vi "Orleen.vi"() -> ()   [LabVIEW 2016]
panel:
  out "String 2":string
  out "Numeric":dbl
  in  "String":string
  in  "?":dbl
  in  "?":dbl
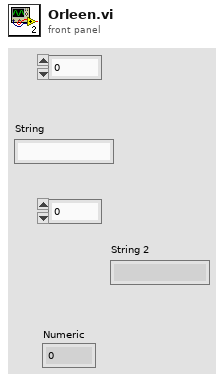
[diagram p1: front panel]
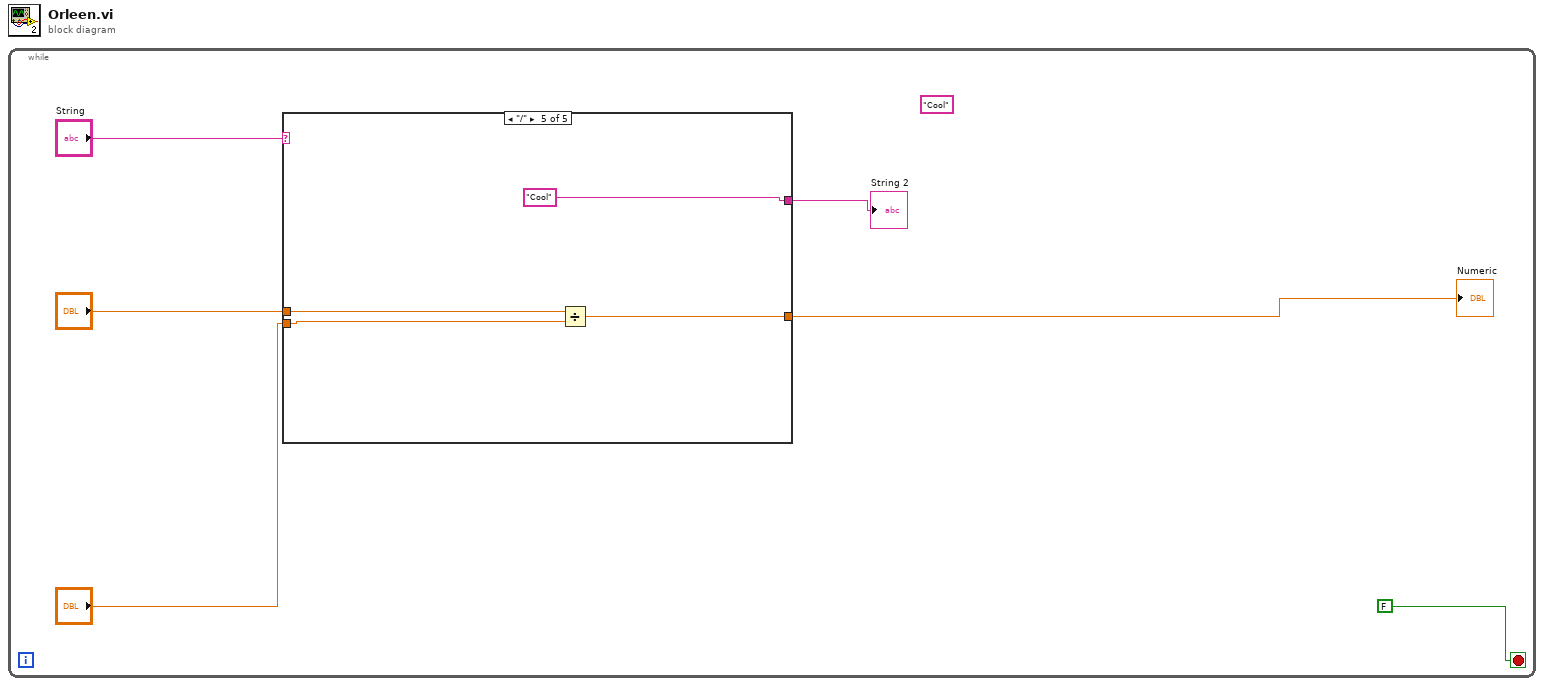
[diagram p0: block diagram]
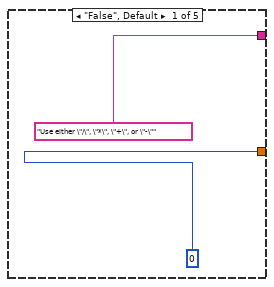
[diagram p2: hidden frame]
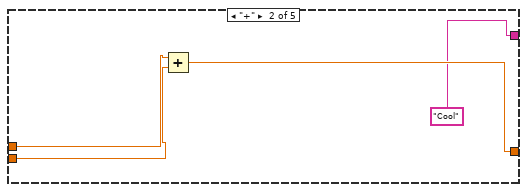
[diagram p3: hidden frame]
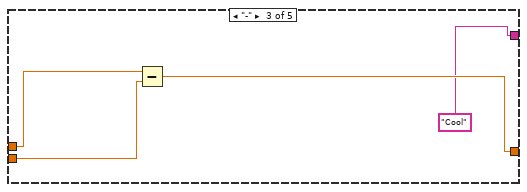
[diagram p4: hidden frame]
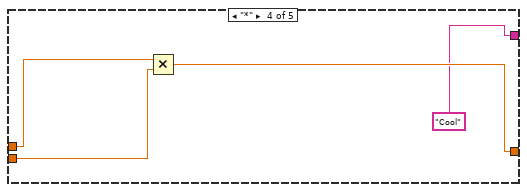
[diagram p5: hidden frame]
diagram:
  n1 = while {
    stop <- FALSE stop-if-true
    (unwired) "Cool"
    n2 = case shown="\"/\"" "String" {
      tunnel: "?" -> [_ w12 w16 w20 w24]
      tunnel: "?" -> [_ w11 w15 w19 w23]
      tunnel: [0 w10 w14 w18 w21] -> w3
      tunnel: ["Use either \"/\", \"*\", \"+\", or \"-\"" "Cool" "Cool" "Cool" "Cool"] -> w2
      frame "False", Default {
      }
      frame "+" {
        n3 = Add(x=w12, y=w11) -> (x+y=w10:dbl)
      }
      frame "-" {
        n4 = Subtract(x=w16, y=w15) -> (x-y=w14:dbl)
      }
      frame "*" {
        n5 = Multiply(x=w20, y=w19) -> (x*y=w18:dbl)
      }
      frame "/" {
        n6 = Divide(x=w24, y=w23) -> (x/y=w21:dbl)
      }
    }
    "Numeric" <- w3
    "String 2" <- w2
  }
